vi "NI VeriStand - Open Custom Device Reference.vi"(8 "error in (no error)":errorcluster, 10 "Gateway IP Address (\"\": localhost)":string, 11 "Custom Device Path":string) -> (0 "error out":errorcluster, 3 "Custom Device":T1)   [LabVIEW 2020, in "NI_VS Custom Device ExecutionAPI.lvlib"]
doc: "Opens a reference to a custom device that you can use to send messages to the custom device. You can use the reference this VI returns with other Custom Device Communication VIs."
uses:
  <vilib>/NI VeriStand/Execution/CustomDevice/NI_VS Custom Device ExecutionAPI.lvlib
  <vilib>/NI VeriStand/Execution/CustomDevice/Custom Device Ref.ctl
  NationalInstruments.VeriStand.ClientAPI
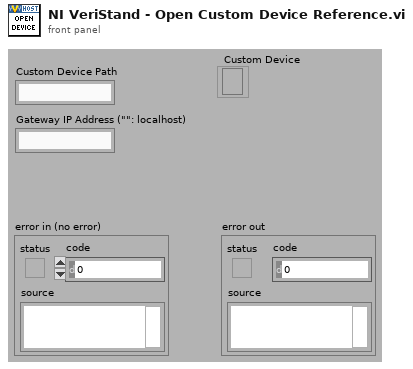
[diagram p1: front panel]
types:
  T1 = typedef "NI_VS Custom Device ExecutionAPI.lvlib/Custom Device Ref.ctl" = refnum<k24>
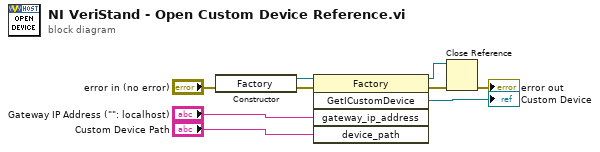
[diagram p0: block diagram]
diagram:
  n1 = constructor class="Factory"(error in="error in (no error)") -> (reference out=w9:refnum<k24>, error out=w8:errorcluster)  [unwired: 2 in, 1 out]
  n2 = invoke class="Factory" method="GetICustomDevice"(reference=w9, error in=w8, "gateway_ip_address"="Gateway IP Address (\"\": localhost)", "device_path"="Custom Device Path") -> (reference out=w3:refnum<k24>, error out=w4:errorcluster, "GetICustomDevice"=→"Custom Device":refnum<k24>)  [unwired: 1 in, 2 out]
  n3 = Close Reference(reference=w3, error in (no error)=w4) -> (error out=→"error out":errorcluster)
